vi "loadControls.vi"(7 "prevName":string caption="default name", 8 "error in (no error)":errorcluster, 9 "Autoload?":bool, 10 "ControlsToLoad":refnum<vi>[](array[refnum]), 11 "ConfigXMLControls":T1) -> (0 "error out":errorcluster, 3 "nameUsed":string)   [LabVIEW 2015]
uses:
  ConfigXMLControl.ctl
  <vilib>/NI/GXML/_subVIs/GXML SearchParser/Search Parser.vi
  <vilib>/NI/GXML/GXML.lvlib
panel:
  # "Loads the selected controls from an XML file. If autoLoad is selected,\nloads the most recently created autosave file"
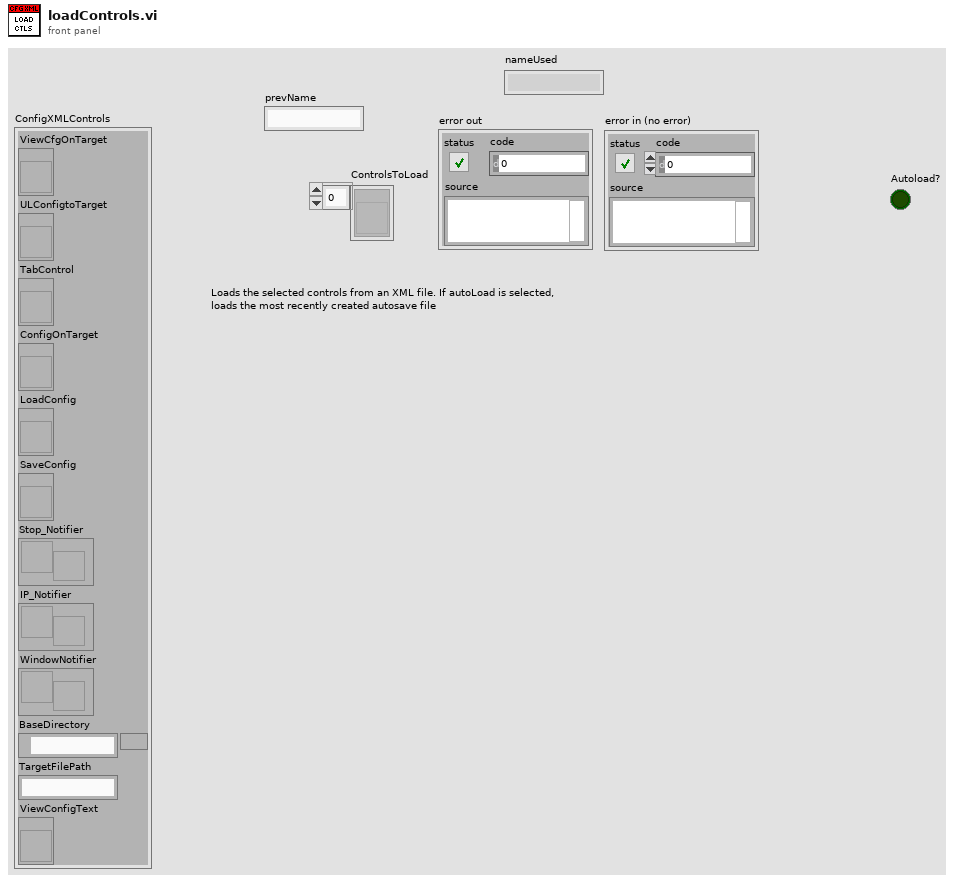
[diagram p1: front panel]
types:
  T1 = typedef "ConfigXMLControl.ctl" = cluster{"ViewCfgOnTarget":refnum<vi>, "ULConfigtoTarget":refnum<vi>, "TabControl":refnum<vi>, "ConfigOnTarget":refnum<vi>, "LoadConfig":refnum<vi>, "SaveConfig":refnum<vi>, "Stop_Notifier":refnum<notifier>, "IP_Notifier":refnum<notifier>, "WindowNotifier":refnum<notifier>, "BaseDirectory":path, "TargetFilePath":string, "ViewConfigText":refnum<vi>}
  T2 = cluster{"appended path":path, "File Created Date (UTC)":timestamp}
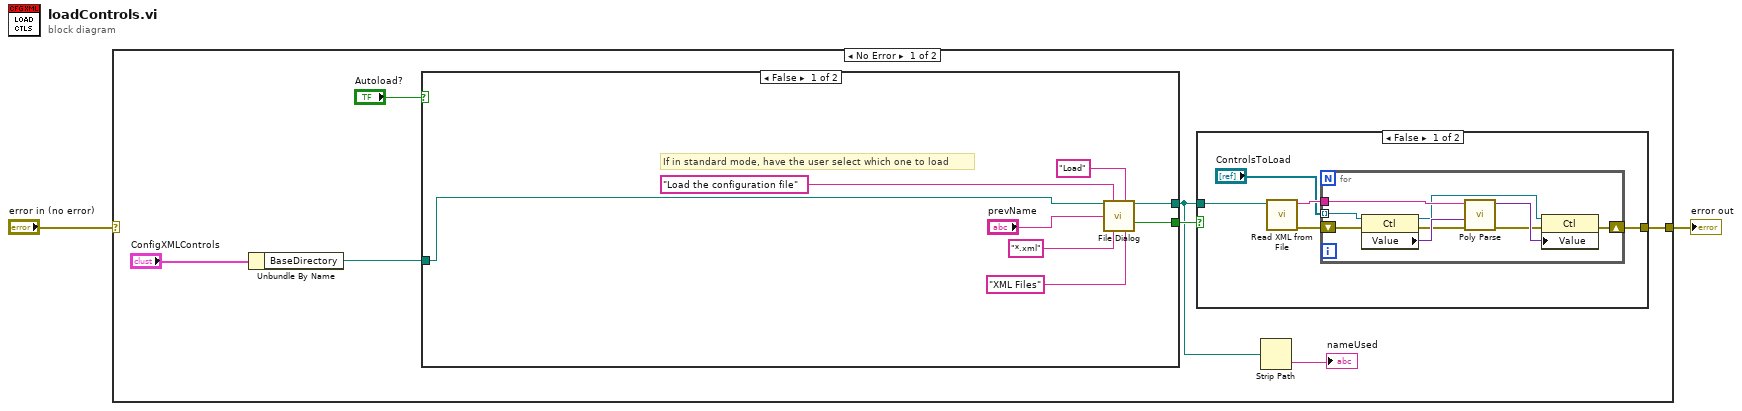
[diagram p0: block diagram]
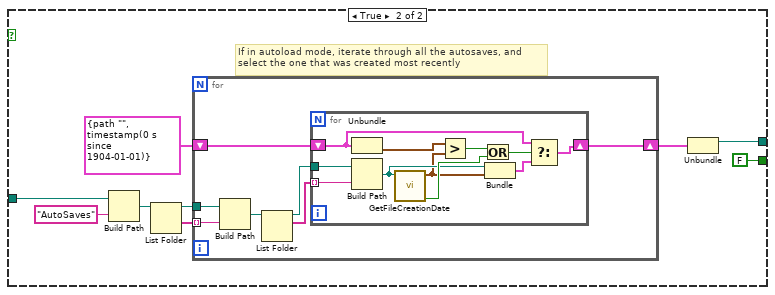
[diagram p3: hidden frame]
diagram:
  n1 = case shown="No Error" "error in (no error)" {
    selector: "error in (no error)" -> [_ w59]
    tunnel: [w5 w59] -> w2
    frame No Error {
      n2 = Unbundle By Name("ConfigXMLControls") -> ("BaseDirectory"=w7:path)
      n3 = case shown="False" "Autoload?" {
        tunnel: w7 -> [w26 w40]
        tunnel: [w24 w33] -> w4
        tunnel: [w25 FALSE ("cancelled")] -> w6
        frame False {
          # "If in standard mode, have the user select which one to load"
          n4 = call "File Dialog"("start path"=w26, "prompt"="Load the configuration file", "button label"="Load", "default name"="prevName", "pattern (all files)"="*.xml", "pattern label"="XML Files") -> ("selected path"=w24:path, "cancelled"=w25:bool)  [unwired: 6 in, 2 out]
        }
        frame True {
          # "If in autoload mode, iterate through all the autosaves, and \nselect the one that was created most recently"
          n5 = Build Path(base path=w40, name or relative path="AutoSaves") -> (appended path=w38:path)
          n6 = List Folder(path=w38) -> (path out=w36:path, folder names=w37:string[])  [unwired: 3 in, 2 out]
          n7 = for {
            tunnel: w37 -> [w45] mode=indexing
            shift-right: [w46] -> w34
            shift-left: cluster{path, timestamp} {path "", timestamp(0 s since 1904-01-01)} -> [w47]
            tunnel: w36 -> [w44]
            n8 = Build Path(base path=w44, name or relative path=w45) -> (appended path=w43:path)
            n9 = List Folder(path=w43) -> (path out=w42:path, filenames=w41:string[])  [unwired: 3 in, 2 out]
            n10 = for {
              shift-right: [w48] -> w46
              shift-left: w47 -> [w49]
              tunnel: w41 -> [w57] mode=indexing
              tunnel: w42 -> [w58]
              n11 = Unbundle(w49) -> (w53:timestamp)  [unwired: 1 out]
              n12 = Build Path(base path=w58, name or relative path=w57) -> (appended path=w52:path)
              n13 = call "GetFileCreationDate.vi"("File Path"=w52) -> ("Error"=w56:bool, "File Created Date (UTC)"=w51:timestamp)  [unwired: 7 in]
              n14 = Greater?(x=w53, y=w51) -> (0:w55:bool)
              n15 = Or(x=w55, y=w56) -> (x .or. y?=w54:bool)
              n16 = Bundle("appended path"=w52, "File Created Date (UTC)"=w51) -> (w50:T2)  [unwired: 1 in]
              n17 = Select(t=w49, s=w54, f=w50) -> (s? t:f=w48:T2)
            }
          }
          n18 = Unbundle(w34) -> (w33:path)  [unwired: 1 out]
        }
      }
      n19 = case shown="False" w6 {
        tunnel: w4 -> [w14 _]
        tunnel: [w10 _] -> w5
        frame False {
          n20 = call <vilib>:"Read XML from File.vi"("XML File Path"=w14) -> ("error out"=w11:errorcluster, "XML String Out"=w13:string)  [unwired: 9 in]
          n21 = for {
            tunnel: w13 -> [w23]
            tunnel: "ControlsToLoad" -> [w22] mode=indexing
            shift-right: [w15] -> w10
            shift-left: w11 -> [w16]
            n22 = property class="Ctl"(reference=w22, error in=w16) -> (reference out=w19:refnum<vi>, error out=w18:errorcluster, "Value"=w21:variant)
            n23 = call-poly <vilib>:"Poly Parse.vi"("error in"=w18, "TypeDesc"=w21, "XML String In"=w23) -> ("error out"=w17:errorcluster, "Parsed Data"=w20:variant)  [unwired: 7 in]
            n24 = property class="Ctl"(reference=w19, error in=w17, "Value"=w20) -> (error out=w15:errorcluster)  [unwired: 1 out]
          }
        }
        frame True {
          # "If true, do not load the controls"
        }
      }
      n25 = Strip Path(path=w4) -> (name=→"nameUsed":string)  [unwired: 1 out]
    }
    frame Error {
    }
  }
  "error out" <- w2
